vi "Write DAQ Parameters.vi"(8 "error in (no error)":errorcluster, 10 "DAQ Parameters":T1, 11 "ATS9462 Class in":refnum<class "ATS9462 Class.lvclass">) -> (0 "error out":errorcluster, 3 "ATS9462 Class out":refnum<class "ATS9462 Class.lvclass">)   [LabVIEW 2015, in "ATS9462 Class.lvclass"]
uses:
  ATS9462 Class.lvclass
  DAQ Parameters.ctl
  Trigger Source.ctl
  Trigger Slope.ctl
  Type Defs/OCT DAQ Channel Data Type.ctl
  Clock Control.ctl
  ATS-VI/ATS_ctl/ATS_Global.ctl
  ATS-VI/ATS_ctl/Record.ctl
  ATS-VI/ATS_ctl/Clock.ctl
  ATS-VI/ATS_ctl/ClockSource.ctl
  ATS-VI/ATS_ctl/ClockRate.ctl
  ATS-VI/ATS_ctl/ClockEdge.ctl
  ATS-VI/ATS_ctl/InputCtrl.ctl
  ATS-VI/ATS_ctl/Coupling.ctl
  ATS-VI/ATS_ctl/Range.ctl
  ATS-VI/ATS_ctl/Impedance.ctl
  ATS-VI/ATS_ctl/Bandwidth.ctl
  ATS-VI/ATS_ctl/Trigger.ctl
  ATS-VI/ATS_ctl/TriggerOperation.ctl
  ATS-VI/ATS_ctl/TriggerEngine.ctl
  ATS-VI/ATS_ctl/ExtTrigger.ctl
  ATS-VI/ATS_ctl/ExtTrigRange.ctl
  ATS-VI/ATS_ctl/ATS_Async_Ctrl.ctl
  ATS-VI/ATS_ctl/ATS_Async_Mode.ctl
  ATS-VI/ATS_ctl/ATS_ReadSamples.ctl
  ATS-VI/ATS_ctl/ATS_Async_Setting.ctl
  ATS9462 Class.lvclass/ATS9462 Class.ctl
  ATS-VI/ATS_ctl/ATS_DMA_Channel.ctl
  DAQ Class.lvclass
panel:
  out "Return Code":u32
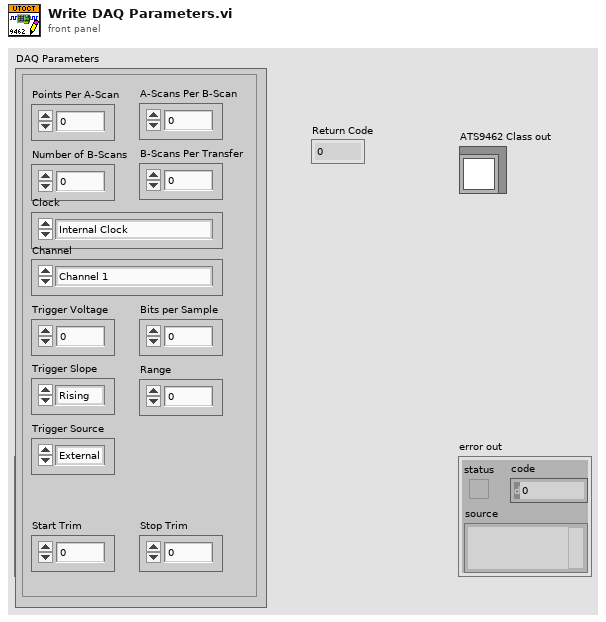
[diagram p1: front panel]
types:
  T1 = typedef "DAQ Class.lvclass/DAQ Parameters.ctl" = cluster{"Points Per A-Scan":u32, "A-Scans Per B-Scan":u32, "Number of B-Scans":u32, "B-Scans Per Transfer":u32, "Trigger Voltage":sgl, "Trigger Source":T2, "Trigger Slope":T3, "Channel":T4, "Clock":T5, "Bits per Sample":dbl, "Range":dbl, "Start Trim":u32, "Stop Trim":u32}
  T2 = typedef "DAQ Class.lvclass/Trigger Source.ctl" = enum16{"External", "Channel A", "Channel B"}
  T3 = typedef "DAQ Class.lvclass/Trigger Slope.ctl" = enum16{"Rising", "Falling"}
  T4 = typedef "OCT DAQ Channel Data Type.ctl" = enum16{"Channel 1", "Channel 2", "Channel 1 and 2"}
  T5 = typedef "DAQ Class.lvclass/Clock Control.ctl" = enum16{"Internal Clock", "External Clock"}
  T6 = typedef "ClockRate.ctl" = u32
  T7 = typedef "ATS_Async_Setting.ctl" = cluster{"UseHeader":u32, "Rec/Buffer":u32, "Total_Rec":u32, "DataBuffer":bool, "GetProcessedData":bool}
  T8 = typedef "ATS_ReadSamples.ctl" = cluster{"Offset":i32, "Length":u32}
  T9 = typedef "ATS_Async_Mode.ctl" = enum16{"Continuous", "Triggered", "No-Pre-Trigger", "Traditional"}
  T10 = typedef "ATS_Async_Ctrl.ctl" = enum16{"SetupDMA", "StartCapture", "Get", "Get_Stream", "Abort", "Stop"}
  T11 = typedef "ATS_Global.ctl" = cluster{"Record":T12, "Clock":T13, "Input A":T16, "Input B":T16, "Trigger":T21}
  T12 = typedef "Record.ctl" = cluster{"Count":u32, "Presize":u32, "Length":u32}
  T13 = typedef "Clock.ctl" = cluster{"ClckSource":T14, "ClckRate":T6, "ClckEdge":T15, "Decimation":u32}
  T14 = typedef "ClockSource.ctl" = enum16{"Internal", "External", "Medium Ext.", "Slow Ext.", "Ext. AC", "Ext. DC", "Ext. (PLL)"}
  T15 = typedef "ClockEdge.ctl" = u16
  T16 = typedef "InputCtrl.ctl" = cluster{"Coupling":T17, "Range":T18, "Impedance":T19, "Bandwidth":T20}
  T17 = typedef "Coupling.ctl" = enum16{"AC", "DC"}
  T18 = typedef "Range.ctl" = u32
  T19 = typedef "Impedance.ctl" = enum16{"1M ohms", "50 ohms"}
  T20 = typedef "Bandwidth.ctl" = enum16{"Full Bandwidth", "Reduce Bandwidth"}
  T21 = typedef "Trigger.ctl" = cluster{"TrigOperation":T22, "Timeout (s)":dbl, "Trig. Delay":u32, "Engine X":T23, "Engine Y":T23, "ExtTrigControl":T24}
  T22 = typedef "TriggerOperation.ctl" = enum16{"Only X", "Only Y", "X or Y", "X and Y", "X xor Y", "X and not Y", "not X and Y"}
  T23 = typedef "TriggerEngine.ctl" = cluster{"Source":enum32{"Chan_A", "Chan_B", "External", "Disable"}, "Slope":enum32{"Positive", "Negative"}, "Level":u32}
  T24 = typedef "ExtTrigger.ctl" = cluster{"Coupling":T17, "Range":T25}
  T25 = typedef "ExtTrigRange.ctl" = enum16{"1 V", "5 V", "TTL"}
  T26 = enum32{"Chan_A", "Chan_B", "External", "Disable"}
  T27 = typedef "ATS_DMA_Channel.ctl" = enum16{"Channel_A", "Channel_B", "A & B"}
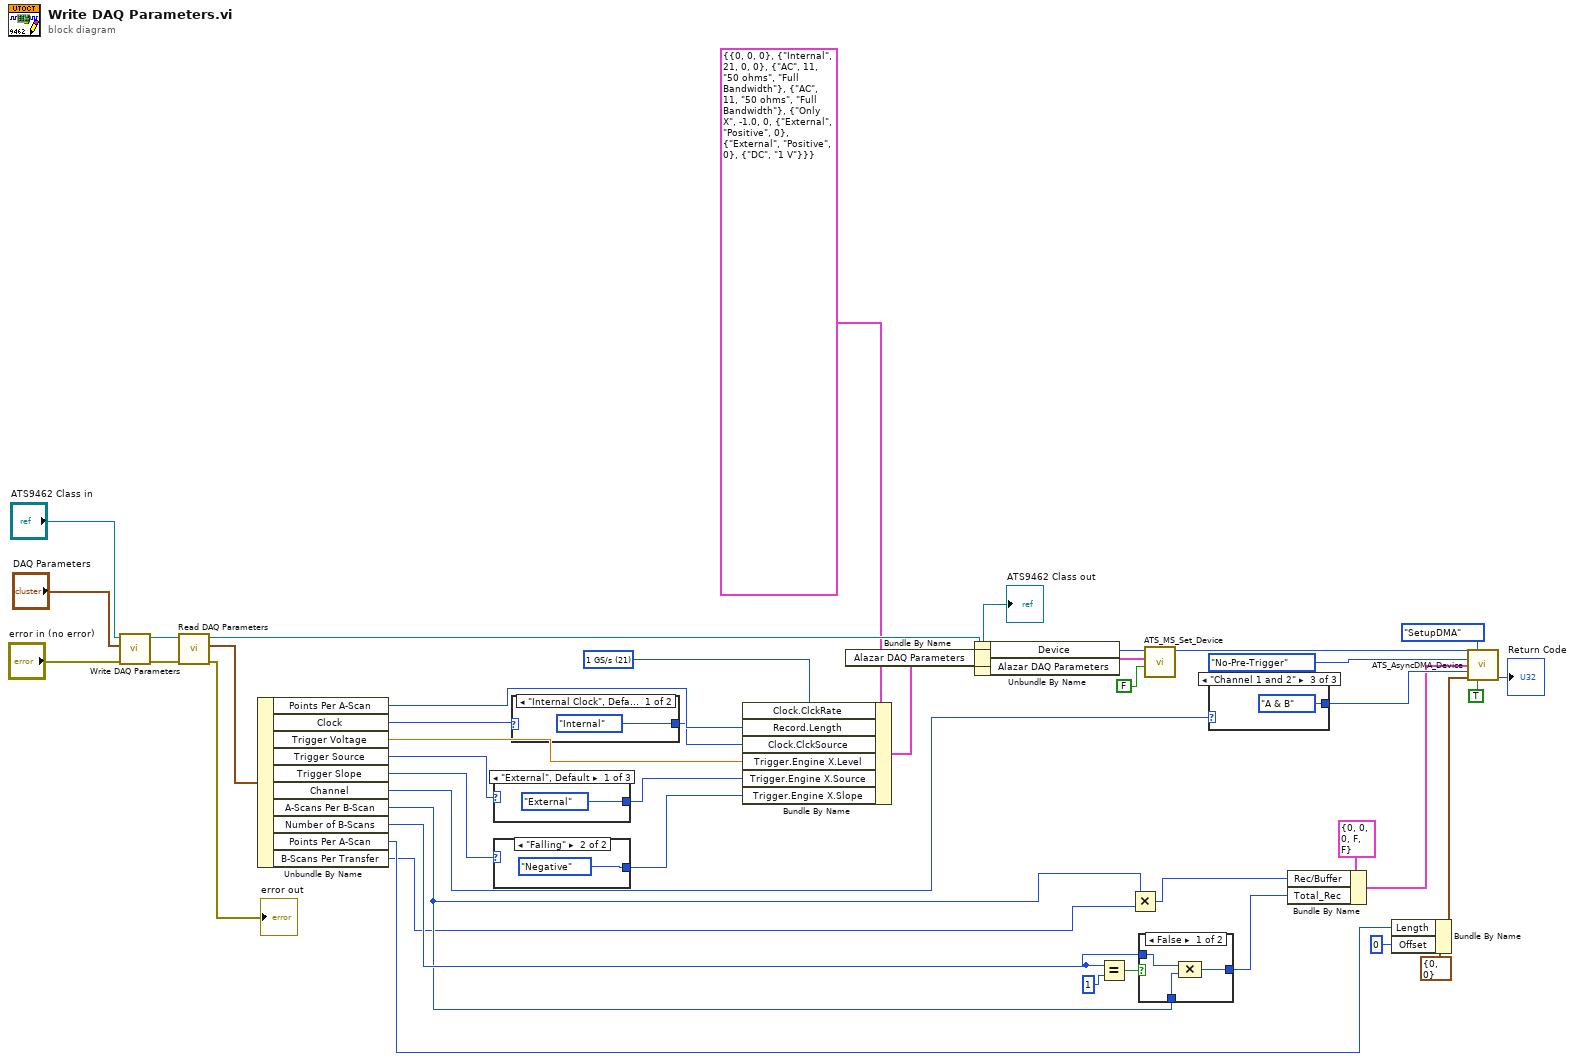
[diagram p0: block diagram]
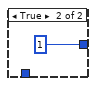
[diagram p2: hidden frame]
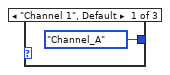
[diagram p3: hidden frame]
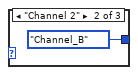
[diagram p4: hidden frame]
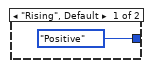
[diagram p5: hidden frame]
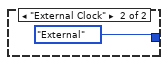
[diagram p6: hidden frame]
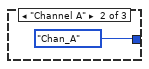
[diagram p7: hidden frame]
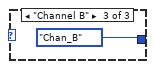
[diagram p8: hidden frame]
diagram:
  w9 = T6 21 items=["1 kS/s", "2 kS/s", "5 kS/s", "10 kS/s", "20 kS/s", "50 kS/s", "100 kS/s", "200 kS/s", "500 kS/s", "1 MS/s", "2 MS/s", "5 MS/s", "10 MS/s", "20 MS/s", "25 MS/s", "50 MS/s", "100 MS/s", "125 MS/s", "200 MS/s", "250 MS/s", "500 MS/s", "1 GS/s"] ("Clock.ClckRate")
  n1 = call-parent "Write DAQ Parameters.vi"("error in (no error)"="error in (no error)", "DAQ Parameters"="DAQ Parameters", "DAQ Class in"="ATS9462 Class in") -> ("error out"=w39:errorcluster, "DAQ Class out"=w40:refnum<class "ATS9462 Class.lvclass">)  [unwired: 7 in]
  n2 = call-dynamic "Read DAQ Parameters.vi"("error in (no error)"=w39, "ATS9462 Class in"=w40) -> ("error out"=→"error out":errorcluster, "DAQ Parameters"=w38:T1, "ATS9462 Class out"=w31:refnum<class "ATS9462 Class.lvclass">)  [unwired: 7 in]
  n3 = Unbundle By Name(w38) -> ("Points Per A-Scan"=w35:u32, "Clock"=w34:T5, "Trigger Voltage"=w32:sgl, "Trigger Source"=w37:T2, "Trigger Slope"=w30:T3, "Channel"=w22:T4, "A-Scans Per B-Scan"=w2:u32, "Number of B-Scans"=w5:u32, "Points Per A-Scan"=w11:u32, "B-Scans Per Transfer"=w1:u32)
  n4 = case shown="\"External\", Default" w37 {
    tunnel: [T26."External" ("Trigger.Engine X.Source") T26."Chan_A" ("Trigger.Engine X.Source") T26."Chan_B" ("Trigger.Engine X.Source")] -> w36
    frame "External", Default {
    }
    frame "Channel A" {
    }
    frame "Channel B" {
    }
  }
  n5 = case shown="\"Falling\"" w30 {
    tunnel: [enum32{"Positive", "Negative"}."Positive" ("Trigger.Engine X.Slope") enum32{"Positive", "Negative"}."Negative" ("Trigger.Engine X.Slope")] -> w29
    frame "Rising", Default {
    }
    frame "Falling" {
    }
  }
  n6 = case shown="\"Internal Clock\", Default" w34 {
    tunnel: [ClockSource."Internal" ("Clock.ClckSource") ClockSource."External" ("Clock.ClckSource")] -> w33
    frame "Internal Clock", Default {
    }
    frame "External Clock" {
    }
  }
  n7 = Bundle By Name(cluster=T11 {"Record"={"Count"=0, "Presize"=0, "Length"=0}, "Clock"={"ClckSource"=enum."Internal", "ClckRate"=21, "ClckEdge"=0, "Decimation"=0}, "Input A"={"Coupling"=enum."AC", "Range"=11, "Impedance"=enum."50 ohms", "Bandwidth"=enum."Full Bandwidth"}, "Input B"={"Coupling"=enum."AC", "Range"=11, "Impedance"=enum."50 ohms", "Bandwidth"=enum."Full Bandwidth"}, "Trigger"={"TrigOperation"=enum."Only X", "Timeout (s)"=-1.0, "Trig. Delay"=0, "Engine X"={"Source"=enum."External", "Slope"=enum."Positive", "Level"=0}, "Engine Y"={"Source"=enum."External", "Slope"=enum."Positive", "Level"=0}, "ExtTrigControl"={"Coupling"=enum."DC", "Range"=enum."1 V"}}} ("Value"), "Clock.ClckRate"=w9, "Record.Length"=w35, "Clock.ClckSource"=w33, "Trigger.Engine X.Level"=w32, "Trigger.Engine X.Source"=w36, "Trigger.Engine X.Slope"=w29) -> (w21:T11)
  n8 = Bundle By Name(cluster=w31, "Alazar DAQ Parameters"=w21) -> (w15:refnum<class "ATS9462 Class.lvclass">)
  "ATS9462 Class out" <- w15
  n9 = Unbundle By Name(w15) -> ("Device"=w19:i32, "Alazar DAQ Parameters"=w18:T11)
  n10 = Equal?(x=w5, y=u32 1) -> (x = y?=w7:bool)
  n11 = Multiply(x=w2, y=w1) -> (x*y=w3:u32)
  n12 = case shown="False" w7 {
    tunnel: [w53 u32 1 ("y")] -> w6
    tunnel: w5 -> [w52 _]
    tunnel: w2 -> [w51 _]
    frame False {
      n13 = Compound Arithmetic op=MULTIPLY(w52, w51) -> (w53:u32)
    }
    frame True {
    }
  }
  n14 = call "ATS_MS_Set_Device.vi"("Set_Manually (F)"=FALSE, "Setup_In"=w18, "DeviceIn"=w19) -> ("DeviceOut"=w16:i32)  [unwired: 3 in, 5 out]
  n15 = case shown="\"Channel 1 and 2\"" w22 {
    tunnel: [ATS_DMA_Channel."Channel_A" ("Channel") ATS_DMA_Channel."Channel_B" ("Channel") ATS_DMA_Channel."A & B" ("Channel")] -> w28
    frame "Channel 1", Default {
    }
    frame "Channel 2" {
    }
    frame "Channel 1 and 2" {
    }
  }
  n16 = Bundle By Name(cluster=T7 {"UseHeader"=0, "Rec/Buffer"=0, "Total_Rec"=0, "DataBuffer"=FALSE, "GetProcessedData"=FALSE} ("Async_Setting"), "Rec/Buffer"=w3, "Total_Rec"=w6) -> (w13:T7)
  n17 = Bundle By Name(cluster=T8 {"Offset"=0, "Length"=0} ("ReadSamples"), "Length"=w11, "Offset"=0) -> (w26:T8)
  n18 = call "ATS_AsyncDMA_Device.vi"("DeviceIn"=w16, "ATS_Async_Ctrl"=ATS_Async_Ctrl."SetupDMA" ("ATS_DMA_Ctrl"), "Async_Mode"=ATS_Async_Mode."No-Pre-Trigger", "Async_Setting"=w13, "Channel"=w28, "ReadSamples"=w26, "Start Now / Wait"=TRUE) -> ("Return Code"=→"Return Code":u32)  [unwired: 4 in, 4 out]
